vi "Read meas.valid.vi"(11 "sync.resources":T1) -> (2 "meas.valid":bool, 3 "sync.resources":T1)   [LabVIEW 2015, in "ni579x Synchronization v1 FPGA.lvlib"]
uses:
  <instrlib>/ni579x/Synchronization/v1/FPGA/ni579x Synchronization v1 FPGA.lvlib
  <instrlib>/ni579x/Synchronization/v1/FPGA/Implementation/Resources.ctl
  <vilib>/rvi/DataTransferAndStorage/Container/Common/niFpgaContainerExecOnDevCompGetState.vi
  <vilib>/rvi/Emulation/niFpgaEmulationIsFPGAContextNoSignature.vi
  <vilib>/rvi/DataTransferAndStorage/Container/Common/niFpgaContainerGetUniqueNameForEmu.vi
  <vilib>/rvi/Memory/Memory_Emulation/niFpgaMemoryEmulationCacheClearOnFirstRun.vi
  <vilib>/rvi/Memory/Memory_Emulation/nirvimemoryEmulationManagerCache_MakeExclusive.vi
  <vilib>/rvi/Memory/Memory_Emulation/niFpgaMemoryEmulationValidateCache.vi
  <vilib>/rvi/Memory/Memory_Emulation/nirvimemoryEmulationManagerCache_InsertValue.vi
  <vilib>/Utility/error.llb/Clear Errors.vi
  <vilib>/rvi/Memory/Memory_Emulation/nirvimemoryEmulationManagerCache_ReleaseExclusive.vi
  <vilib>/rvi/Memory/Memory_Emulation/nirvimemoryEmulationManagerCache_GetValue.vi
  <vilib>/rvi/Memory/Memory_Emulation/nirvimemoryEmulationManagerCache_SetValue.vi
  <vilib>/rvi/Emulation/niFpgaProcessEmulError.vi
  <vilib>/rvi/Emulation/niFpgaSctlEmulationGetInTimedLoop.vi
  <vilib>/rvi/DataTransferAndStorage/Container/XNode/niFpgaContainer.xnode
  <vilib>/rvi/DataTransferAndStorage/Register/Emulation/niFpgaRegisterEmulationRefIn.vi
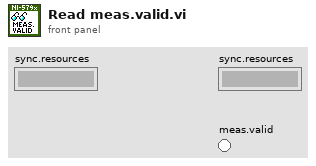
[diagram p1: front panel]
types:
  T1 = typedef "ni579x Synchronization v1 FPGA.lvlib/Resources.ctl" = cluster{"master":refnum<k21>, "meas.enable":refnum<k21>, "meas.ready":refnum<k21>, "meas.arm":refnum<k21>, "meas.valid":refnum<k21>, "meas.value":refnum<k21>, "meas.oversample clock":refnum<k21>, "meas.oversample factor":refnum<k21>, "cptr":refnum<k21>, "cptr.adjust":refnum<k21>, "cptr.period":refnum<k21>}
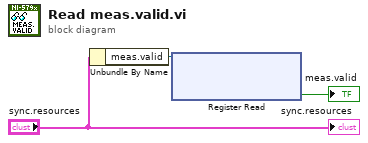
[diagram p0: block diagram]
diagram:
  n1 = Unbundle By Name("sync.resources") -> ("meas.valid"=w3:refnum<k21>)
  n2 = xnode ("Register Read")("Register In"=w3) -> ("Data"=→"meas.valid":bool)  [unwired: 1 out]
  "sync.resources" <- "sync.resources"
